vi "G2131-i仪器串口通讯11111.vi"(0 "VISA resource name":refnum<visa-resource-name>="COM3", 2 "baud rate (9600)":u32=9600) -> (1 "Delta2Min":string, 5 "H2O":string, 6 "12CO2":string, 7 "12CO2(dry）":string, 8 "Delta5Min":string, 9 "13CO2":string, 10 "13CO2（dry）":string)   [LabVIEW 2016]
uses:
  <vilib>/Instr/_visa.llb/VISA Configure Serial Port (Instr).vi
panel:
  out "返回数 2":u32
  out "read buffer":string
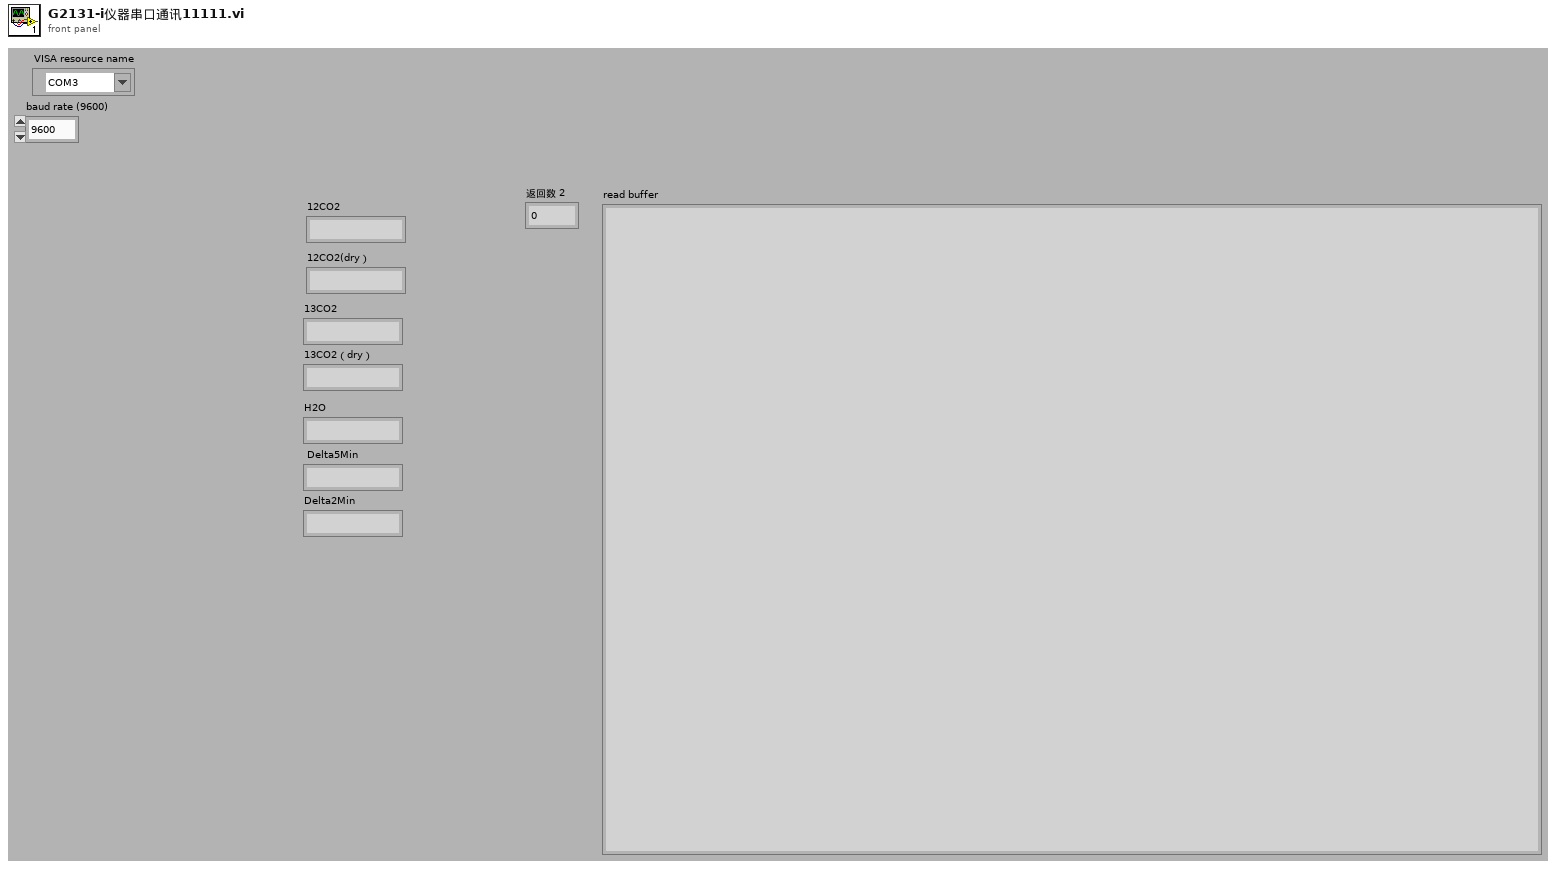
[diagram p1: front panel]
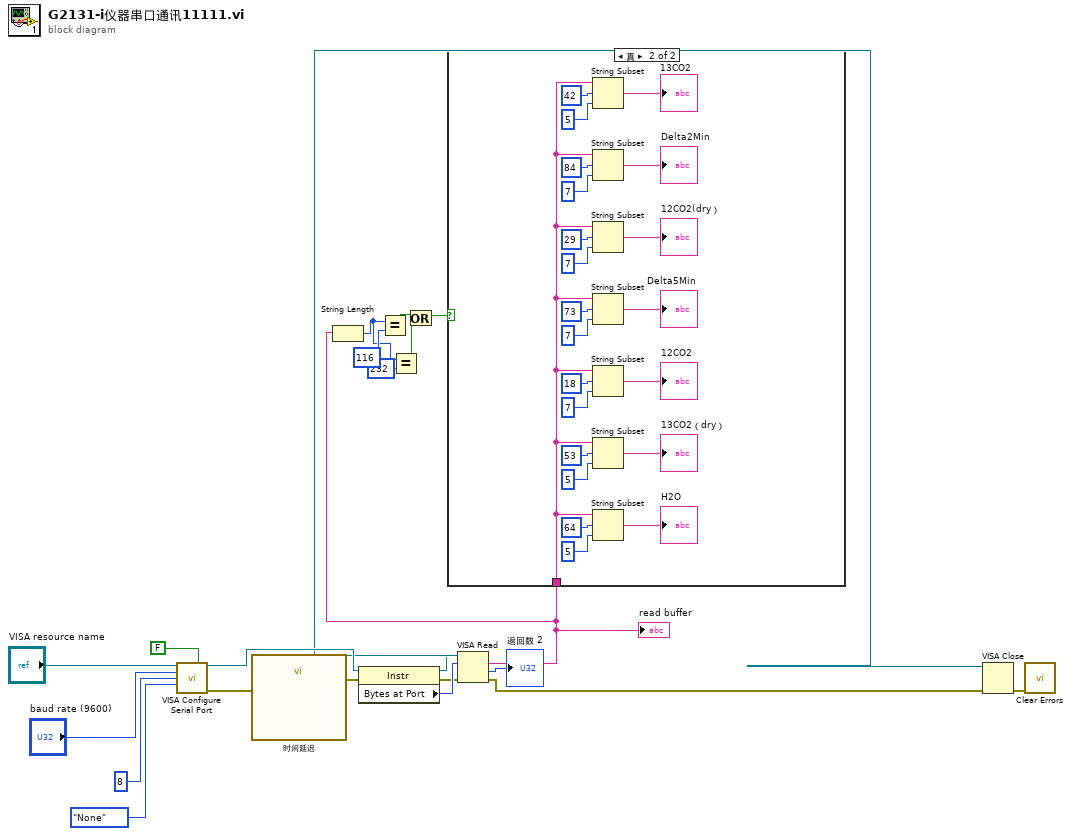
[diagram p0: block diagram]
diagram:
  n1 = call-poly "VISA Configure Serial Port"("VISA resource name"="VISA resource name", "Enable Termination\nChar (T)"=FALSE ("Enable Termination\nChar (T)"), "baud rate (9600)"="baud rate (9600)", "data bits (8)"=u16 8, "parity (0:none)"=enum16{"None", "Odd", "Even", "Mark", "Space"}."None") -> ("VISA resource name out"=w19:refnum<visa-resource-name>, "error out"=w18:errorcluster)  [unwired: 9 in]
  n2 = call "时间延迟"("error in (no error)"=w18) -> ("error out"=w12:errorcluster)  [unwired: 10 in]
  n3 = property class="Instr"(reference=w19, error in=w12) -> (reference out=w9:refnum<visa-resource-name>, error out=w10:errorcluster, "Bytes at Port"=w11:u32)
  n4 = VISA Read(VISA resource name=w9, byte count=w11, error in (no error)=w10) -> (VISA resource name out=w16:refnum<visa-resource-name>, read buffer=w7:string, return count=→"返回数 2":u32, error out=w17:errorcluster)
  "read buffer" <- w7
  n5 = String Length(string=w7) -> (length=w4:i32)
  n6 = Equal?(x=w4, y=116) -> (x = y?=w2:bool)
  n7 = Equal?(x=w4, y=232) -> (x = y?=w1:bool)
  n8 = Or(x=w2, y=w1) -> (x .or. y?=w5:bool)
  n9 = case shown="真" w5 {
    tunnel: w7 -> [_ w29]
    frame False {
    }
    frame True {
      n10 = String Subset(string=w29, offset (0)=42 ("偏移量(0)"), length (rest)=5 ("长度（剩余）")) -> (substring=→"13CO2":string)
      n11 = String Subset(string=w29, offset (0)=84 ("偏移量(0)"), length (rest)=7 ("长度（剩余）")) -> (substring=→"Delta2Min":string)
      n12 = String Subset(string=w29, offset (0)=29 ("偏移量(0)"), length (rest)=7 ("长度（剩余）")) -> (substring=→"12CO2(dry）":string)
      n13 = String Subset(string=w29, offset (0)=73 ("偏移量(0)"), length (rest)=7 ("长度（剩余）")) -> (substring=→"Delta5Min":string)
      n14 = String Subset(string=w29, offset (0)=18 ("偏移量(0)"), length (rest)=7 ("长度（剩余）")) -> (substring=→"12CO2":string)
      n15 = String Subset(string=w29, offset (0)=53 ("偏移量(0)"), length (rest)=5 ("长度（剩余）")) -> (substring=→"13CO2（dry）":string)
      n16 = String Subset(string=w29, offset (0)=64 ("偏移量(0)"), length (rest)=5 ("长度（剩余）")) -> (substring=→"H2O":string)
    }
  }
  n17 = VISA Close(VISA resource name=w16, error in (no error)=w17) -> (error out=w13:errorcluster)
  n18 = call <vilib>:"Clear Errors.vi"("error in (no error)"=w13) -> ()  [unwired: 5 in, 2 out]
